vi "MATLAB script node - Lorenz Diff Eq.vi"() -> ()   [LabVIEW 2023]
doc: "Demonstrates how to use m-file script in the MATLAB script node. This VI solves a Lorenz Attractor differential equation using m-file script and plots the resulting Lorenz Attractor. The MathWorks, Inc. MATLAB (R) Application Software version 5.0 or later must be installed in order to run this VI."
uses:
  <vilib>/Math Plots/3D Math Plots/3D Comet/3D Comet XCtrl/3D Comet.xctl
  <vilib>/Math Plots/3D Math Plots/3D Comet/3D Comet Datatype/Public/Plot Helper (Vector).vi
  <vilib>/Math Plots/3D Math Plots/3D Comet/3D Comet Datatype/3D Comet Datatype.lvclass
panel:
  out "3D Comet":refnum<class "3D Plot Datatype.lvclass">[](xcontrol)
  out "Lorenz Attractor":cluster{"t":dbl[], "Y":dbl[]}[](graph)
  # "Overview: Solves a Lorenz Attractor differential equation using the MATLAB script node and plots the resulting Lorenz Attractor.\nRequirements: LabVIEW Full Development System, The MathWorks, Inc. MATLAB (R) Application Software version 5.0 or later\nInstructions: \nRun the VI."
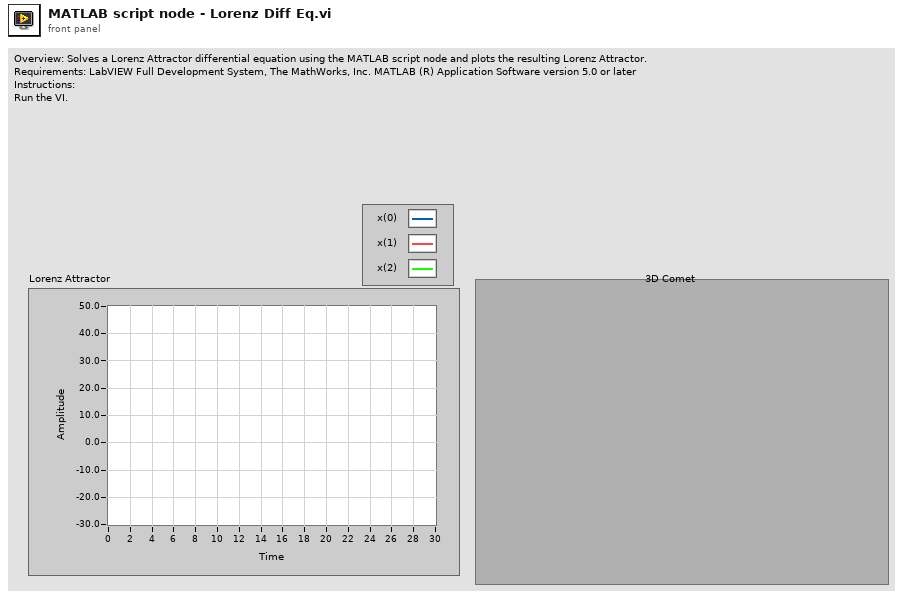
[diagram p1: front panel]
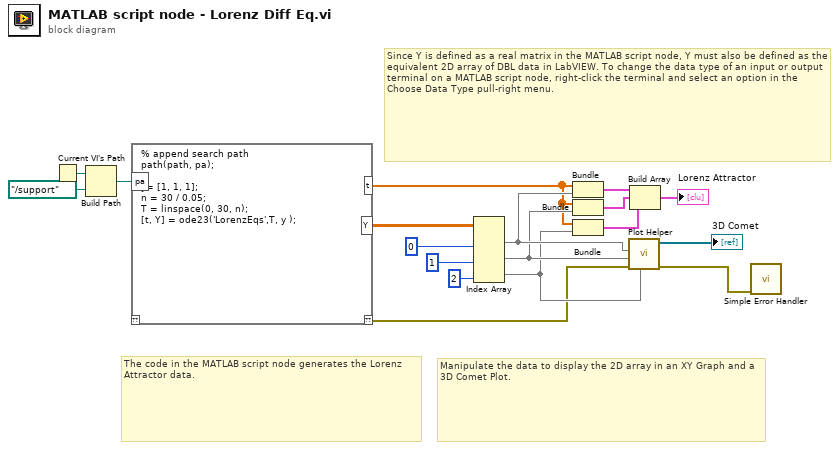
[diagram p0: block diagram]
diagram:
  # "Manipulate the data to display the 2D array in an XY Graph and a 3D Comet Plot."
  # "The code in the MATLAB script node generates the Lorenz Attractor data."
  # "Since Y is defined as a real matrix in the MATLAB script node, Y must also be defined as the equivalent 2D array of DBL data in LabVIEW. To change the data type of an input or output terminal on a MATLAB script node, right-click the terminal and select an option in the Choose Data Type pull-right menu."
  n1 = Current VI's Path() -> (path=w6:path)
  n2 = Build Path(base path=w6, name or relative path=path "../support") -> (appended path=w4:path)
  n3 = script code="% append search path\npath(path, pa);\n\ny= [1, 1, 1];\nn = 30 / 0.05;\nT = linspace(0, 30, n);\n[t, Y] = ode23('LorenzEqs',T, y );"("pa"=w4) -> ("??"=w1:errorcluster, "t"=w3:dbl[], "Y"=w2:dbl[][])  [unwired: 1 in]
  n4 = Index Array(array=w2, index (col) #1=0 ("disabled index (col)"), index (col) #2=1 ("index (col)"), index (col) #3=2 ("index (col)")) -> (element #1=w14:dbl[], element #2=w12:dbl[], element #3=w10:dbl[])  [unwired: 3 in]
  n5 = Bundle(w3, w14) -> (w13:cluster{dbl[], dbl[]})  [unwired: 1 in]
  n6 = Bundle(w3, w12) -> (w11:cluster{dbl[], dbl[]})  [unwired: 1 in]
  n7 = Bundle(w3, w10) -> (w9:cluster{dbl[], dbl[]})  [unwired: 1 in]
  n8 = call-poly <vilib>:"Plot Helper.vi"("z vector"=w10, "error in (no error)"=w1, "y vector"=w12, "x vector"=w14) -> ("error out"=w7:errorcluster, "3D Plot lvclass Array out"=→"3D Comet":refnum<class "3D Plot Datatype.lvclass">[])  [unwired: 2 in, 4 out]
  n9 = Build Array(w13, w11, w9) -> (→"Lorenz Attractor":cluster{dbl[], dbl[]}[])
  n10 = call <vilib>:"Simple Error Handler.vi"("error in (no error)"=w7) -> ()  [unwired: 4 in, 5 out]
